vi "AlliGator Add New Gate to Array, Sum , Min & Max Image.vi"(0 "SGL Gate Images in":T1[](array[typedef]), 1 "Buffer Image Available":bool, 5 "SGL Image Max in":T1, 7 "SGL Image Sum in":T1, 9 "SGL Image Min in":T1, 11 "error in (no error)":errorcluster, 12 "Gate Image":T1, 13 "Current Gate":i32) -> (4 "SGL Gate Images out":T1[](array[typedef]), 6 "SGL Image Max out":T1, 8 "SGL Image Sum out":T1, 10 "SGL Image Min out":T1, 15 "error out":errorcluster)   [LabVIEW 2021, in "AlliGator Files.lvlib"]
doc: "Adds the new <B>Gate Image</b> to the gate image array and use it to build the Min, Max and Sum images."
uses:
  AlliGator Files.lvlib
  <vilib>/vision/Image Controls.llb/IMAQ Image.ctl
  <vilib>/vision/NI_Vision_Development_Module.lvlib
  Image/Image.lvlib
panel:
  # "see the AlliGator License on the block diagram (Ctrl+E or Window:Show Block Diagram)"
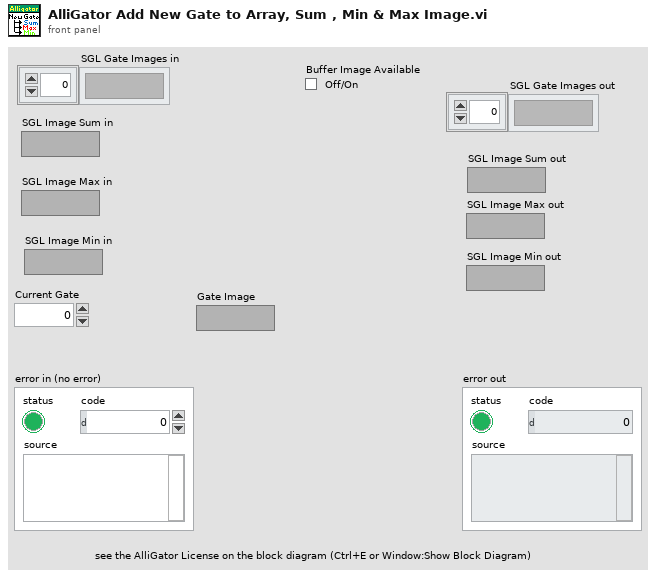
[diagram p1: front panel]
types:
  T1 = typedef "IMAQ Image.ctl" = refnum<image>
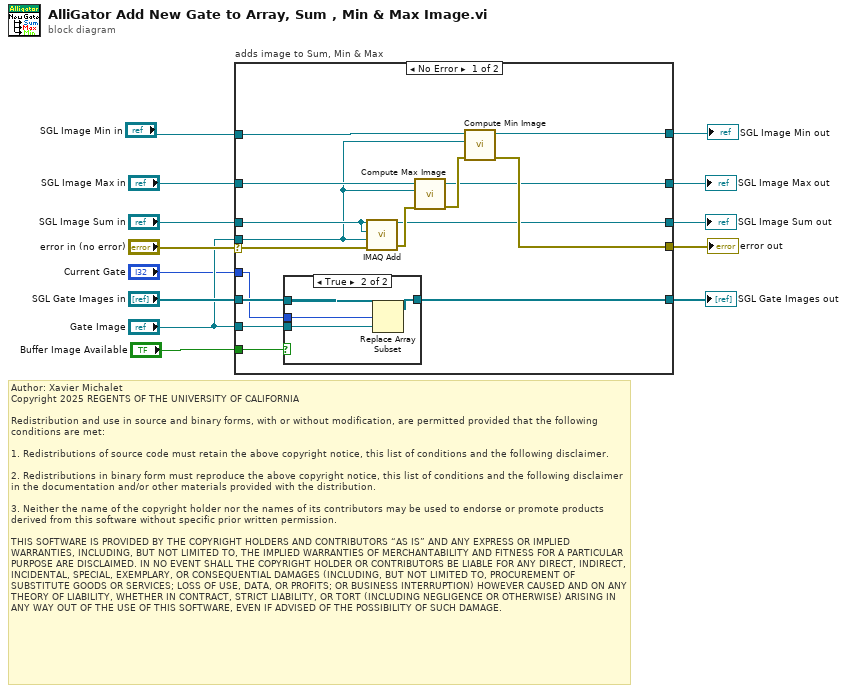
[diagram p0: block diagram]
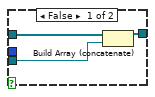
[diagram p2: hidden frame]
diagram:
  # "Author: Xavier Michalet\nCopyright 2025 REGENTS OF THE UNIVERSITY OF CALIFORNIA\n\nRedistribution and use in source and binary forms, with or without modification, are permitted provided that the following conditions are met:\n\n1. Redistributions of source code must retain the above copyright notice, this list of conditions and the following disclaimer.\n\n2. Redistributions in binary form must reproduce the above copyright notice, this list of conditions and the following disclaimer in the documentation and/or other materials provided with the distribution.\n\n3. Neither the name of the copyright holder nor the names of its contributors may be used to endorse or promote products derived from this software without specific prior written permission.\n\nTHIS SOFTWARE IS PROVIDED BY THE COPYRIGHT HOLDERS AND CONTRIBUTORS “AS IS” AND ANY EXPRESS OR IMPLIED WARRANTIES, INCLUDING, BUT NOT LIMITED TO, THE IMPLIED WARRANTIES OF MERCHANTABILITY AND FITNESS FOR A PARTICULAR PURPOSE ARE DISCLAIMED. IN NO EVENT SHALL THE COPYRIGHT HOLDER OR CONTRIBUTORS BE LIABLE FOR ANY DIRECT, INDIRECT, INCIDENTAL, SPECIAL, EXEMPLARY, OR CONSEQUENTIAL DAMAGES (INCLUDING, BUT NOT LIMITED TO, PROCUREMENT OF SUBSTITUTE GOODS OR SERVICES; LOSS OF USE, DATA, OR PROFITS; OR BUSINESS INTERRUPTION) HOWEVER CAUSED AND ON ANY THEORY OF LIABILITY, WHETHER IN CONTRACT, STRICT LIABILITY, OR TORT (INCLUDING NEGLIGENCE OR OTHERWISE) ARISING IN ANY WAY OUT OF THE USE OF THIS SOFTWARE, EVEN IF ADVISED OF THE POSSIBILITY OF SUCH DAMAGE."
  n1 = case "adds image to Sum, Min & Max" shown="No Error" "error in (no error)" {
    selector: "error in (no error)" -> [w23 w37]
    tunnel: "SGL Image Sum in" -> [w22 w41]
    tunnel: "Gate Image" -> [w19 _]
    tunnel: [w14 w41] -> w6
    tunnel: [w17 w37] -> w4
    tunnel: "Gate Image" -> [w27 _]
    tunnel: "Buffer Image Available" -> [w29 _]
    tunnel: "SGL Gate Images in" -> [w28 w40]
    tunnel: "Current Gate" -> [w25 _]
    tunnel: [w26 w40] -> w7
    tunnel: "SGL Image Max in" -> [w24 w39]
    tunnel: [w15 w39] -> w9
    tunnel: "SGL Image Min in" -> [w20 w38]
    tunnel: [w16 w38] -> w1
    frame No Error {
      n2 = case shown="True" w29 {
        tunnel: w28 -> [w32 w36]
        tunnel: w27 -> [w31 w35]
        tunnel: w25 -> [_ w33]
        tunnel: [w30 w34] -> w26
        frame False {
          n3 = Build Array (concatenate)(w32, w31) -> (w30:T1[])
        }
        frame True {
          n4 = Replace Array Subset(array=w36, new element=w35, index=w33) -> (w34:T1[])
        }
      }
      n5 = call "IMAQ Add"("Image Src A"=w22, "Image Dst"=w22, "Image Src B"=w19, "error in (no error)"=w23) -> ("Image Dst Out"=w14:T1, "error out"=w21:errorcluster)  [unwired: 3 in]
      n6 = call "Compute Max Image.vi"("error in (no error)"=w21, "New Image"=w19, "Max Image Dst"=w24) -> ("error out"=w18:errorcluster, "Max Image"=w15:T1)  [unwired: 7 in]
      n7 = call "Compute Min Image.vi"("error in (no error)"=w18, "New Image"=w19, "Min Image Dst"=w20) -> ("error out"=w17:errorcluster, "Min Image"=w16:T1)  [unwired: 7 in]
    }
    frame Error {
    }
  }
  "SGL Image Max out" <- w9
  "SGL Gate Images out" <- w7
  "SGL Image Sum out" <- w6
  "error out" <- w4
  "SGL Image Min out" <- w1
